vi "battery Profile.vi"() -> ()   [LabVIEW 2015]
uses:
  <instrlib>/Agilent N6700 Series/Agilent N6700 Series.lvlib
panel:
  out "error out 3":errorcluster
  out "error out":errorcluster
  out "Ver":string
  out "error out 2":errorcluster
  in  "Data Log Period (s)":dbl=1.0 format="%#_13g"
  in  "VISA resource name":refnum<visa-resource-name>="VAL_N6705B"
  in  "Number Of DUT":i32=1
  in  "Reset Time (S) \nAfter Discharging":u32
  in  "Number Of Cycle\n(Charching & Discharching For Each DUT":i32=1
  in  "Test Machine IP":string="192.168.1.200"
  in  "Stop":bool
  out "Control Value:Get All":cluster{"Name":string, "Variant Data":variant}[](array[cluster])
  in  "Save":bool
  in  "Start":bool
  out "Status":string
  out "Time 2":dbl caption="Time(s)" format="%#.0f"
  in  "Sleep (s)":u32=3000
  out "Curent Tracking 2":dbl caption="Curent Tracking" format="%.8f"
  out "Voltage Tracking 2":dbl caption="Voltage Tracking" format="%.8f"
  in  "Discharge Stop Voltage":dbl=3.5 format="%#_13g"
  in  "Discharg current Limit":dbl=-0.1 format="%#_13f"
  out "Charging P 2":bool
  out "Charging P 1":bool
  out "Time(s)":u64
  in  "Stop Current(A) after Full":dbl=0.05 format="%#_13g"
  out "Current Tracking":dbl format="%.8f"
  out "Voltage Tracking":dbl format="%.8f"
  in  "Stop Voltage(V)":dbl=4.34 format="%_5f"
  in  "Charge Current (A)":dbl=0.06 format="%#_13g"
  in  "Set Voltge(V)":dbl=4.35 format="%_3f"
  # "Battery Tester"
  # "Battery Charging"
  # "Battery Discharging"
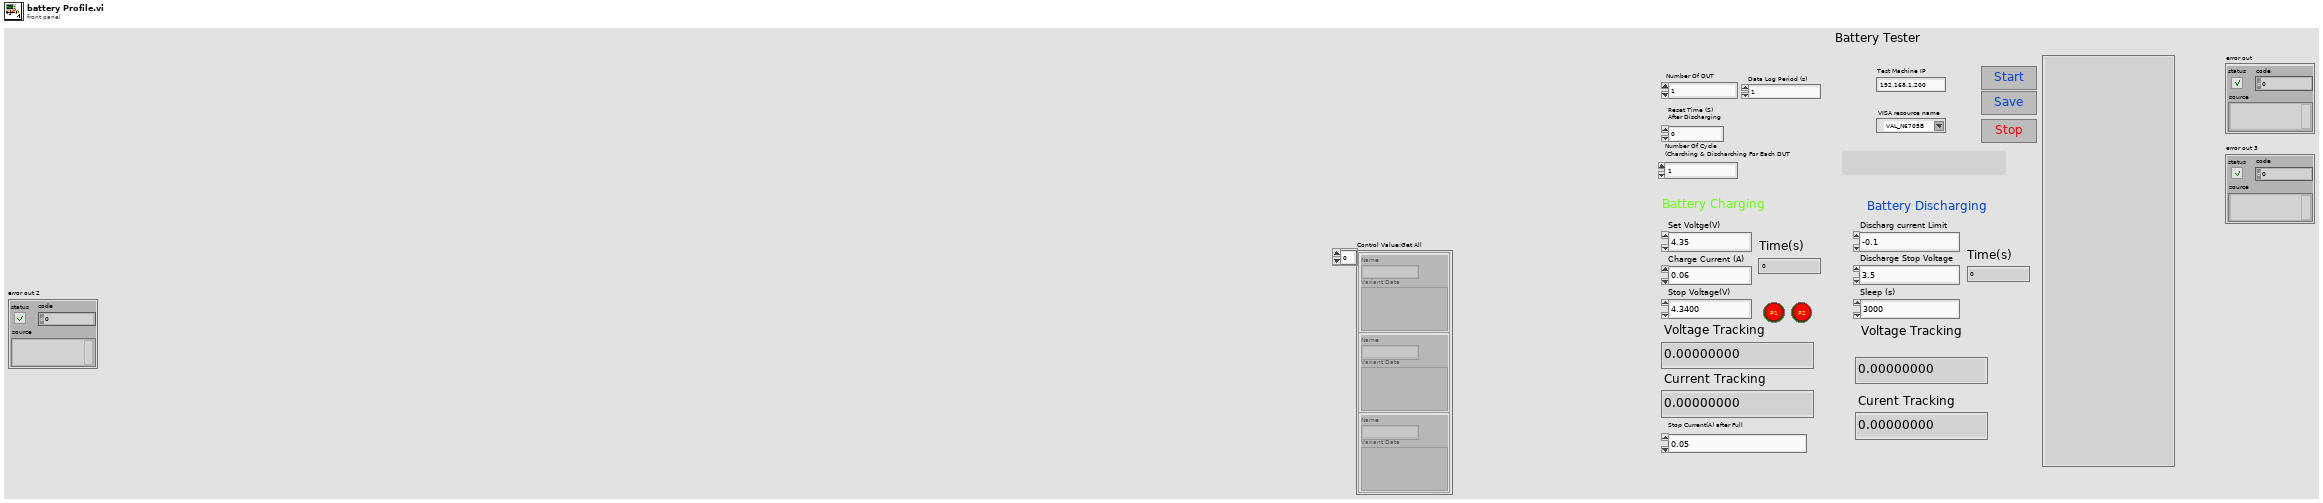
[diagram p1: front panel]
types:
  T1 = enum16{"2 Quad Power Supply", "Unipower Supply", "CC Load", "CV Load", "VM", "CM"}
  T2 = enum16{"open", "replace", "create", "open or create", "replace or create", "replace or create with confirmation"}
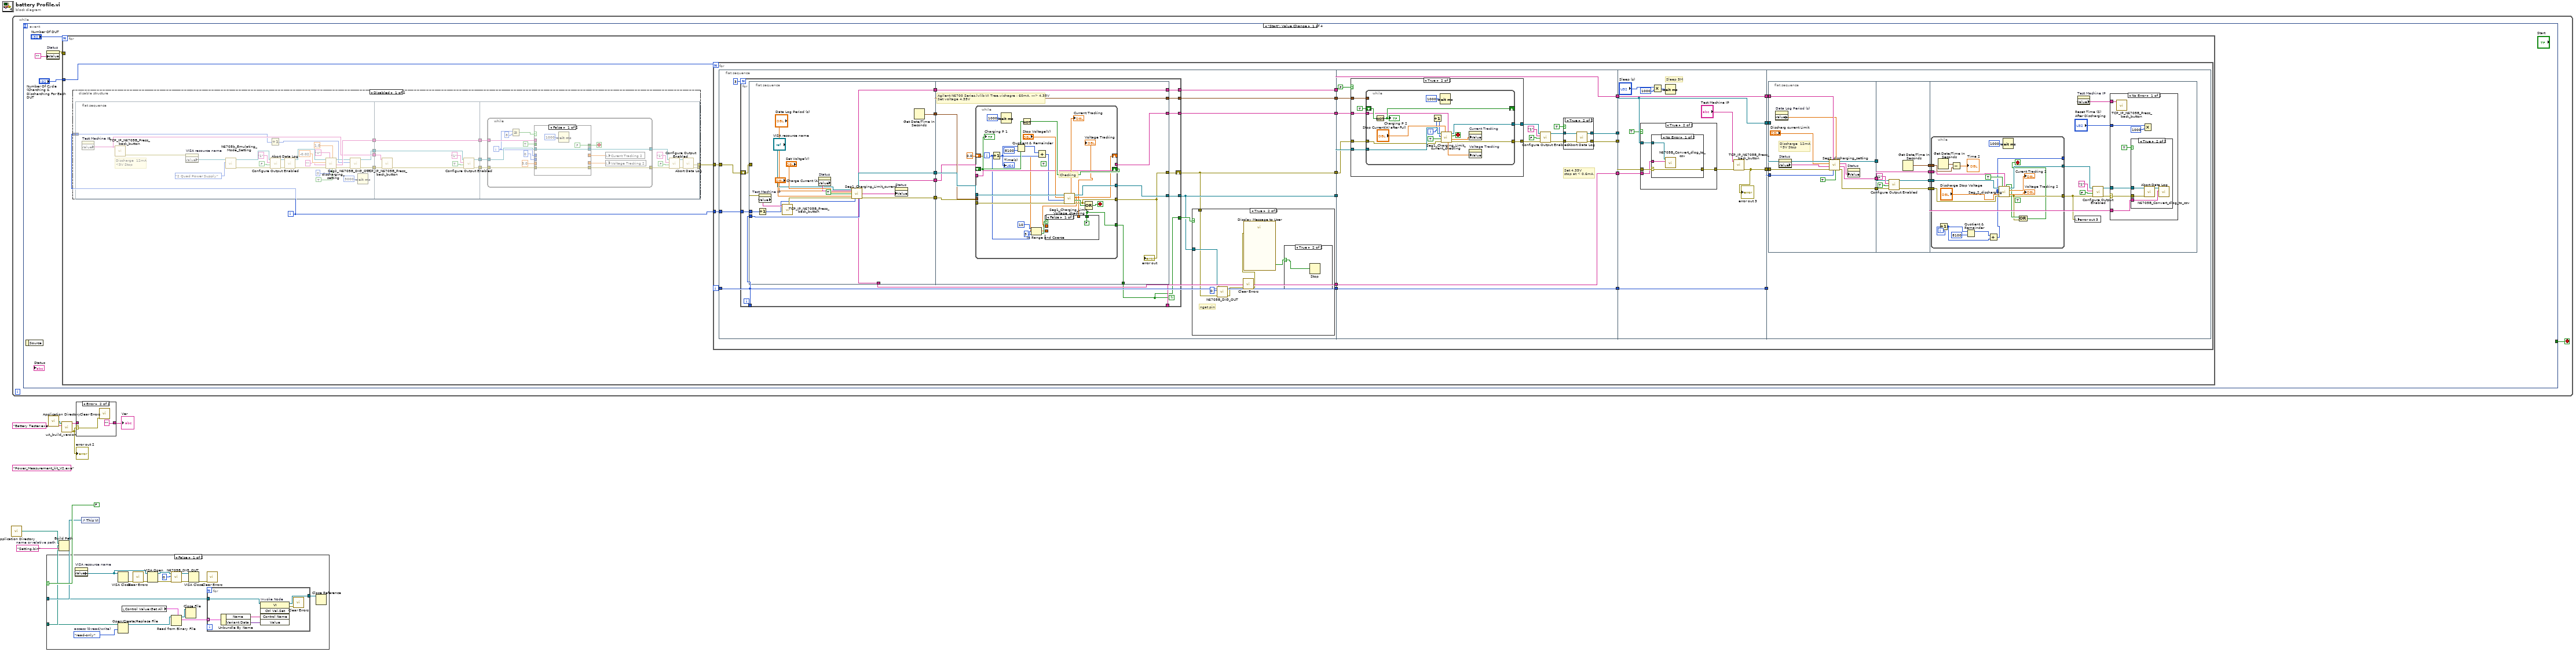
[diagram p0: block diagram]
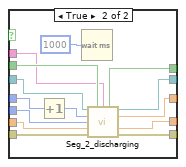
[diagram p3: hidden frame]
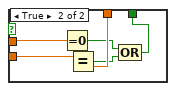
[diagram p7: hidden frame]
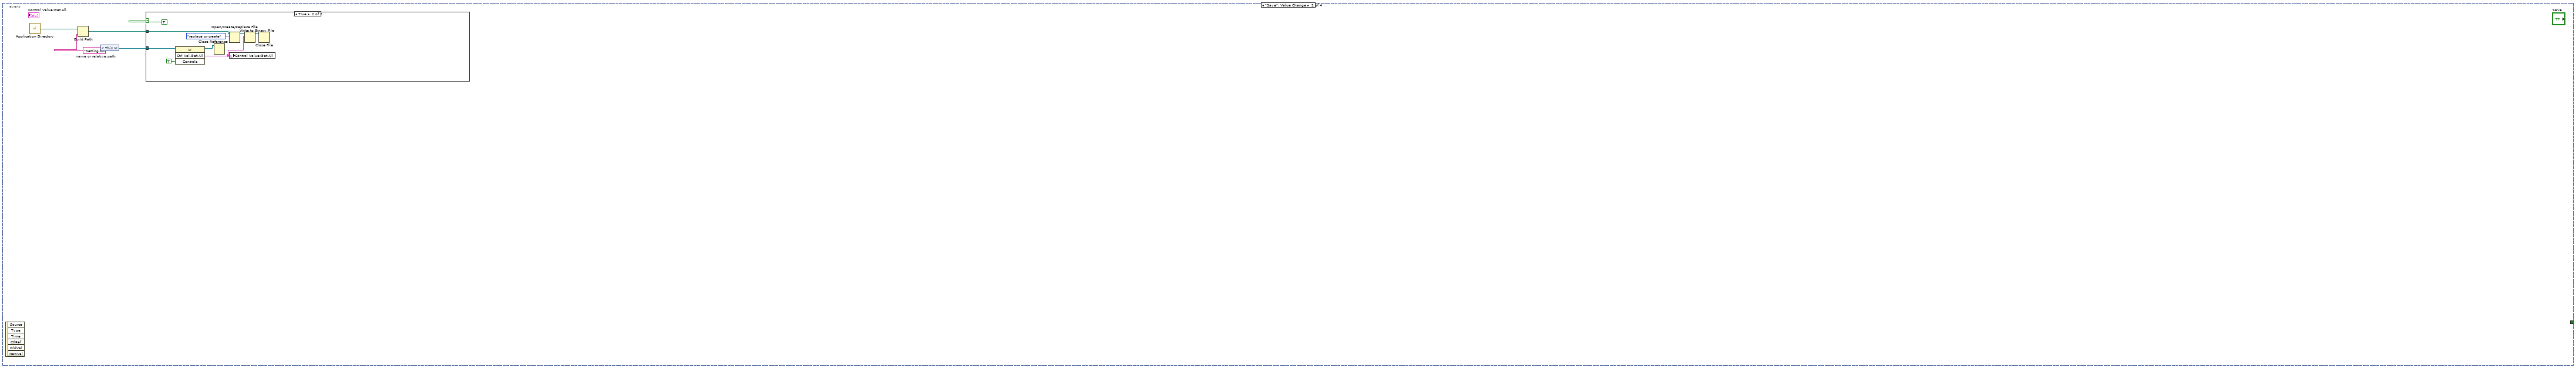
[diagram p14: hidden frame]
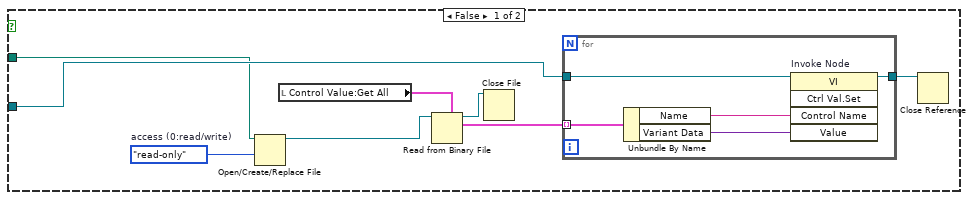
[diagram p15: hidden frame]
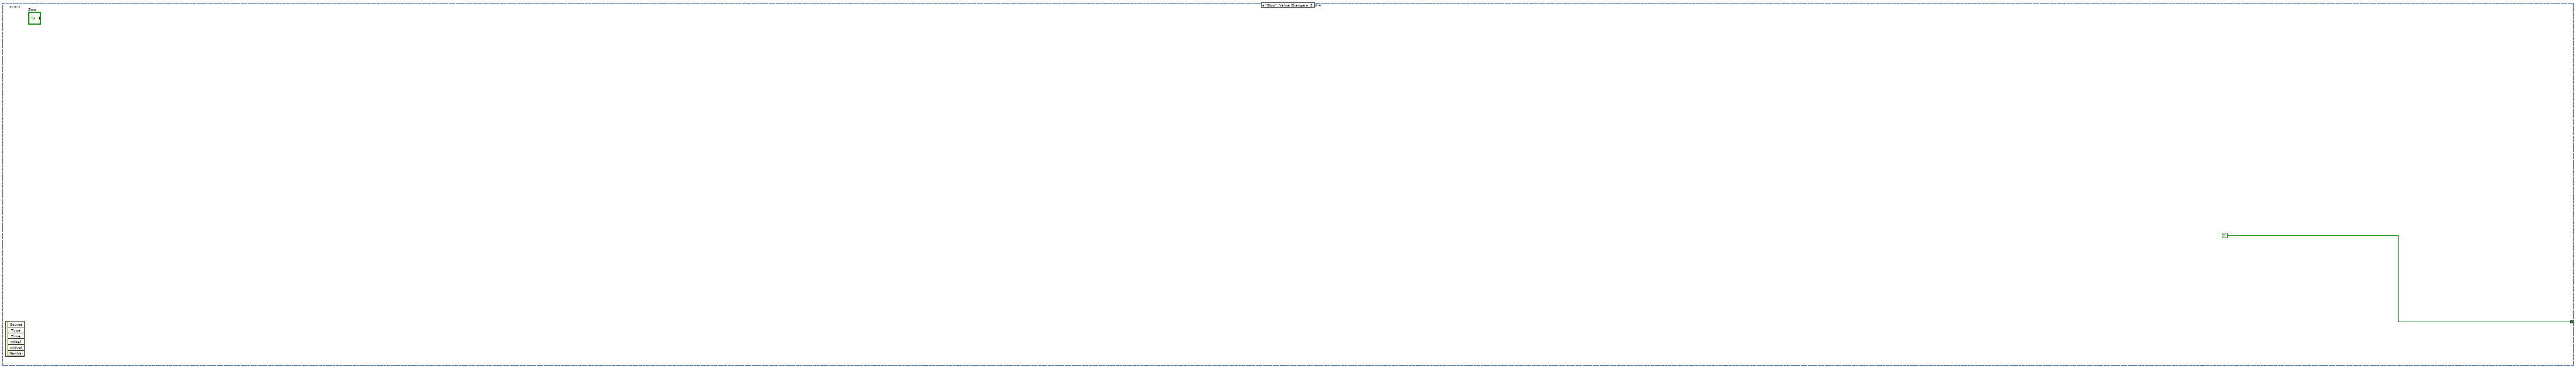
[diagram p16: hidden frame]
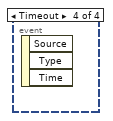
[diagram p17: hidden frame]
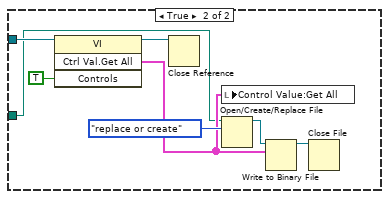
[diagram p18: hidden frame]
diagram:
  (unwired) "Power_Measurement_kit_V2.exe" ("name or relative path")
  w7 = "Setting.bin"  # name or relative path
  n1 = call <vilib>:"Application Directory.vi"() -> ("Application Directory"=w8:path)
  n2 = while {
    stop <- w11 stop-if-true
    n3 = event shown="[0] \"Start\": Value Change" {
      selector: _ -> [_ _ _ _]
      dyn-events: _ -> [_ _ _ _]
      timeout: _ -> [_ _ _ _]
      tunnel: [_ _ TRUE _] -> w11
      event "Start": Value Change {
        n4 = event-data() -> ()  [unwired: 1 in, 1 out]
        n5 = property on="Status" class="Str"("Value"="") -> (error out=w12:errorcluster)  [unwired: 2 in, 1 out]
        n6 = for {
          N: "Number Of DUT" -> [_]
          tunnel: "Number Of Cycle\n(Charching & Discharching For Each DUT" -> [w18]
          tunnel: w12 -> [_]
          i -> [w16]
          n7 = disable-structure shown="Disabled" {
            disable-tunnel: [w20 _] -> w17
            disable-tunnel: w16 -> [w19 _]
            frame Disabled {
              n8 = flat-sequence {
                tunnel: [w32] -> w27
                tunnel: [w31] -> w26
                tunnel: [w52] -> w25
                tunnel: [w34] -> w24
                tunnel: w19 -> [w28]
                tunnel: w27 -> [w60]
                tunnel: w26 -> [w55]
                tunnel: [w59] -> w23
                tunnel: [w58] -> w22
                tunnel: w25 -> [w57]
                tunnel: [w57] -> w21
                tunnel: w24 -> [w54]
                tunnel: w23 -> [w72]
                tunnel: w22 -> [w71]
                tunnel: w21 -> [w65]
                tunnel: [w64] -> w20
                frame #0 {
                  # "Discharge  12mA\n<3V Stop"
                  n9 = property on="Test Machine IP" class="Str"() -> ("Value"=w34:string)  [unwired: 2 in, 2 out]
                  n10 = call "TCP_IP_N6705B_Press_back_button.vi"("instrument address"=w34) -> ("error out"=w46:errorcluster)  [unwired: 10 in]
                  n11 = property on="VISA resource name" class="VISAName"(error in=w46) -> ("Value"=w49:refnum<visa-resource-name>)  [unwired: 1 in, 2 out]
                  n12 = call "N6705b_Emulating_Mode_Setting.vi"("Mode"=T1."2 Quad Power Supply", "VISA resource name"=w49) -> ("error out"=w42:errorcluster, "VISA resource name out"=w44:refnum<visa-resource-name>)  [unwired: 8 in]
                  n13 = Increment(x=w28) -> (x+1=w29:i32)
                  n14 = call <instrlib>:"Configure Output Enabled.vi"("error in (no error)"=w42, "Enable Output (False)"=FALSE, "Channel Name (1)"="1", "VISA resource name"=w44) -> ("error out"=w41:errorcluster, "VISA resource name out"=w43:refnum<visa-resource-name>)  [unwired: 6 in]
                  n15 = call <instrlib>:"Abort Data Log.vi"("error in (no error)"=w41, "VISA resource name"=w43) -> ("error out"=w35:errorcluster, "VISA resource name out"=w45:refnum<visa-resource-name>)  [unwired: 8 in]
                  n16 = call "Seg2_discharging_setting.vi"("Log?"=TRUE, "Data Log Period (0.1 s)"=1.0, "Number of cycles"=0, "N"="X", "error in (no error)"=w35, "Value"="", "Discharg current Limit"=-0.02 ("Discharg current Limit 2"), "VISA Refnum in"=w45) -> ("error out"=w30:errorcluster, "File Name Out"=w52:string, "VISA Refnum out"=w33:refnum<visa-resource-name>)  [unwired: 1 out]
                  n17 = call "N6705B_DIG_OUT.vi"("error in (no error)"=w30, "DUT_1_4"=w29, "VISA Refnum in"=w33) -> ("error out"=w31:errorcluster, "VISA Refnum out"=w32:refnum<visa-resource-name>)  [unwired: 7 in]
                  n18 = Wait (ms)(milliseconds to wait=u32 3000) -> ()  [unwired: 1 out]
                }
                frame #1 {
                  n19 = call "TCP_IP_N6705B_Press_back_button.vi"("error in (no error)"=w55, "instrument address"=w54) -> ("error out"=w56:errorcluster)  [unwired: 9 in]
                  n20 = call <instrlib>:"Configure Output Enabled.vi"("error in (no error)"=w56, "Enable Output (False)"=TRUE, "Channel Name (1)"="1", "VISA resource name"=w60) -> ("error out"=w58:errorcluster, "VISA resource name out"=w59:refnum<visa-resource-name>)  [unwired: 6 in]
                }
                frame #2 {
                  n21 = while {
                    tunnel: w72 -> [w86]
                    tunnel: w71 -> [w85]
                    tunnel: [w84] -> w67
                    tunnel: w65 -> [w80]
                    tunnel: [w73] -> w63
                    i -> [w77]
                    stop <- w83 stop-if-true
                    n22 = Greater Or Equal?(x=w77, y=8) -> (x >= y?=w76:bool)
                    n23 = case shown="False" w76 {
                      tunnel: w86 -> [w89 w104]
                      tunnel: w85 -> [w90 w103]
                      tunnel: [w89 w102] -> w84
                      tunnel: [FALSE ("Stop discharging") w101] -> w83
                      tunnel: 3.0 ("Discharge Stop Voltage 2") -> [_ w100]
                      tunnel: TRUE ("Log??") -> [_ w99]
                      tunnel: w80 -> [_ w98]
                      tunnel: [_ w97] -> w79
                      tunnel: [w90 w96] -> w73
                      tunnel: w77 -> [_ w93]
                      tunnel: 0 ("Index") -> [_ w95]
                      tunnel: [_ w94] -> w74
                      frame False {
                        n24 = Wait (ms)(milliseconds to wait=u32 1000) -> ()  [unwired: 1 out]
                      }
                      frame True {
                        n25 = Increment(x=w93) -> (x+1=w92:i32)
                        n26 = Wait (ms)(milliseconds to wait=u32 1000) -> ()  [unwired: 1 out]
                        n27 = call "Seg_2_discharging.vi"("VISA Refnum in"=w104, "Log??"=w99, "File_name"=w98, "Numeric"=w92, "Index"=w95, "Discharge Stop Voltage"=w100, "error in (no error)"=w103) -> ("Stop discharging"=w101:bool, "VISA Refnum out"=w102:refnum<visa-resource-name>, "Curent Tracking 2"=w94:dbl, "Voltage Tracking 2"=w97:dbl, "error out"=w96:errorcluster)  [unwired: 4 in]
                      }
                    }
                    n28 = local write "Curent Tracking 2"(w74) -> ()
                    n29 = local write "Voltage Tracking 2"(w79) -> ()
                  }
                  n30 = call <instrlib>:"Configure Output Enabled.vi"("error in (no error)"=w63, "Enable Output (False)"=FALSE, "Channel Name (1)"="1", "VISA resource name"=w67) -> ("error out"=w66:errorcluster, "VISA resource name out"=w68:refnum<visa-resource-name>)  [unwired: 6 in]
                  n31 = call <instrlib>:"Abort Data Log.vi"("error in (no error)"=w66, "VISA resource name"=w68) -> ("error out"=w64:errorcluster)  [unwired: 8 in, 1 out]
                }
              }
            }
            frame Enabled {
            }
          }
          n32 = for {
            N: w18 -> [_]
            tunnel: w16 -> [w114]
            tunnel: w17 -> [w106]
            i -> [w112]
            n33 = flat-sequence {
              tunnel: [w125] -> w123
              tunnel: [w124] -> w122
              tunnel: [w134] -> w121
              tunnel: [w133] -> w120
              tunnel: w114 -> [w132]
              tunnel: w112 -> [w131]
              tunnel: [w131] -> w111
              tunnel: [w130] -> w108
              tunnel: w106 -> [w129]
              tunnel: [w128] -> w105
              tunnel: w123 -> [w231]
              tunnel: w122 -> [w230]
              tunnel: [w224] -> w119
              tunnel: [w223] -> w118
              tunnel: w121 -> [w222]
              tunnel: w120 -> [w221]
              tunnel: [w221] -> w117
              tunnel: w111 -> [w219]
              tunnel: [w219] -> w109
              tunnel: w108 -> [w218]
              tunnel: [w218] -> w107
              tunnel: w105 -> [w215]
              tunnel: [w265] -> w116
              tunnel: w119 -> [w265]
              tunnel: w118 -> [w268]
              tunnel: [w270] -> w115
              tunnel: w117 -> [w270]
              tunnel: [w262] -> w113
              tunnel: [w266] -> w110
              tunnel: w109 -> [w266]
              tunnel: w107 -> [w264]
              tunnel: w116 -> [w293]
              tunnel: w115 -> [w287]
              tunnel: w113 -> [w286]
              tunnel: w110 -> [w285]
              frame #0 {
                n34 = for {
                  N: 3 -> [_]
                  tunnel: [w151] -> w125
                  tunnel: [w149] -> w134
                  tunnel: [w148] -> w133
                  tunnel: w132 -> [w147]
                  tunnel: w131 -> [w146]
                  tunnel: [w145] -> w130
                  tunnel: [w143] -> w128
                  shift-right: [w150] -> w124
                  shift-left: w129 -> [w144]
                  tunnel: [w142] -> w126
                  stop <- w142 continue-if-true
                  n35 = flat-sequence {
                    tunnel: [w173] -> w156
                    tunnel: [w172] -> w155
                    tunnel: [w170] -> w154
                    tunnel: [w166] -> w153
                    tunnel: w147 -> [w163]
                    tunnel: w146 -> [w160]
                    tunnel: [w158] -> w145
                    tunnel: [w158] -> w152
                    tunnel: w144 -> [w157]
                    tunnel: w156 -> [w184]
                    tunnel: w155 -> [w183]
                    tunnel: [w182] -> w151
                    tunnel: [w178] -> w150
                    tunnel: w154 -> [w181]
                    tunnel: [w181] -> w149
                    tunnel: w153 -> [w180]
                    tunnel: [w180] -> w148
                    tunnel: w152 -> [w179]
                    tunnel: [w177] -> w143
                    tunnel: [w176] -> w142
                    frame #0 {
                      n36 = Increment(x=w163) -> (x+1=w162:i32)
                      n37 = property on="Test Machine IP" class="Str"(error in=w157) -> ("Value"=w165:string)  [unwired: 1 in, 2 out]
                      n38 = call "TCP_IP_N6705B_Press_back_button.vi"("instrument address"=w165) -> ("error out"=w164:errorcluster)  [unwired: 10 in]
                      n39 = property on="Status" class="Str"() -> ("Value"=w169:string)  [unwired: 2 in, 2 out]
                      n40 = call "Seg1_Charging_Limit_current.vi"("VISA Refnum in"="VISA resource name", "Value"=w169, "Data Log Period (0.1 s)"="Data Log Period (s)", "Set Voltge(V)"="Set Voltge(V)", "Log?"=TRUE, "Charge Current (A)"="Charge Current (A)", "error in (no error)"=w164, "Numeric"=w162, "Number of cycles"=w160) -> ("VISA Refnum out"=w173:refnum<visa-resource-name>, "String"=w166:string, "File Name Out"=w158:string, "String 2"=w168:string, "error out"=w172:errorcluster)  [unwired: 2 in]
                      n41 = property on="Status" class="Str"("Value"=w168) -> ()  [unwired: 2 in, 2 out]
                      n42 = Get Date/Time In Seconds() -> (seconds since 1Jan1904=w170:timestamp)
                    }
                    frame #1 {
                      # "Agilent N6700 Series.lvlib:VI Tree.vichagre : 60mA, ---> 4.35V\nSet voltage 4.35V"
                      n43 = while {
                        tunnel: w184 -> [w207]
                        tunnel: w183 -> [w206]
                        tunnel: [w205] -> w182
                        tunnel: [w195] -> w178
                        tunnel: w181 -> [_]
                        shift-right: [w202] -> _
                        shift-left: _ -> [w203]
                        tunnel: w179 -> [w193]
                        tunnel: [w193] -> w177
                        tunnel: [w185] -> w176
                        shift-right: [w186] -> _
                        shift-left: 0.0 ("Voltage Tracking") -> [w187]
                        i -> [w188]
                        stop <- w194 stop-if-true
                        (unwired) TRUE ("Log?")
                        # "Checking"
                        n44 = Increment(x=w188) -> (x+1=w197:i32)
                        "Time(s)" <- w197
                        n45 = Wait (ms)(milliseconds to wait=u32 1000) -> ()  [unwired: 1 out]
                        n46 = Quotient & Remainder(x=w197, y=8100) -> (x-y*floor(x/y)=w198:i32)  [unwired: 1 out]
                        n47 = Not(x=w203) -> (.not. x?=w202:bool)
                        n48 = In Range and Coerce(upper limit=10 ("y"), x=w188, lower limit=3) -> (In Range?=w189:bool)  [unwired: 1 out]
                        n49 = Add(x=w198, y=w197) -> (x+y=w192:i32)
                        n50 = call "Seg1_Charging_Limit_Voltage_checking.vi"("error in (no error)"=w206, "Numeric"=w192, "Stop Voltage(V)"="Stop Voltage(V)", "VISA Refnum in"=w207) -> ("error out"=w195:errorcluster, "Boolean"=w196:bool, "Voltage Tracking"=w186:dbl, "VISA Refnum out"=w205:refnum<visa-resource-name>, "Current Tracking"=→"Current Tracking":dbl)  [unwired: 3 in]
                        "Voltage Tracking" <- w186
                        n51 = case shown="False" w189 {
                          tunnel: w186 -> [_ w214]
                          tunnel: w187 -> [_ w213]
                          tunnel: w186 -> [_ w212]
                          tunnel: [FALSE w209] -> w185
                          frame False {
                          }
                          frame True {
                            n52 = Equal To 0?(x=w214) -> (x = 0?=w211:bool)
                            n53 = Equal?(x=w213, y=w212) -> (x = y?=w210:bool)
                            n54 = Compound Arithmetic op=OR(w211, w210) -> (w209:bool)
                          }
                        }
                        n55 = Compound Arithmetic op=OR(w195, w196, w185) -> (w194:bool)
                        "Charging P 1" <- w203
                      }
                      "error out" <- w178
                    }
                  }
                }
                n56 = case shown="True" w126 {
                  tunnel: w125 -> [_ w140]
                  tunnel: w124 -> [_ w138]
                  frame False {
                  }
                  frame True {
                    # "ngat pin"
                    n57 = call "N6705B_DIG_OUT.vi"("error in (no error)"=w138, "DUT_1_4"=0, "VISA Refnum in"=w140) -> ("error out"=w139:errorcluster)  [unwired: 7 in, 1 out]
                    n58 = call <vilib>:"Clear Errors.vi"("error in (no error)"=w139) -> ("error out"=w136:errorcluster)  [unwired: 5 in, 1 out]
                    n59 = call "Display Message to User"("error in (no error)"=w136) -> ("OK"=w135:bool)  [unwired: 9 in, 1 out]
                    n60 = case shown="True" w135 {
                      selector: w135 -> [_ w141]
                      frame False {
                      }
                      frame True {
                        n61 = Stop(stop? (T)=w141) -> ()
                      }
                    }
                  }
                }
              }
              frame #1 {
                # "Set 4.35V\nstop at < 0.6mA,"
                n62 = case shown="True" FALSE {
                  tunnel: w231 -> [w239 w246]
                  tunnel: w230 -> [w238 w245]
                  tunnel: [w239 w244] -> w228
                  tunnel: [w238 w243] -> w227
                  tunnel: w222 -> [_ w242]
                  tunnel: w215 -> [_ w240]
                  frame False {
                    # "Anh Nguyen Request Jan 01 2018"
                  }
                  frame True {
                    n63 = while {
                      tunnel: w246 -> [w261]
                      tunnel: w245 -> [w260]
                      tunnel: [w254] -> w244
                      tunnel: [w251] -> w243
                      tunnel: w242 -> [_]
                      shift-right: [w255] -> _
                      shift-left: TRUE -> [w256]
                      tunnel: w240 -> [w247]
                      i -> [w249]
                      stop <- w259 stop-if-true
                      n64 = Not(x=w256) -> (.not. x?=w255:bool)
                      "Charging P 2" <- w255
                      n65 = Increment(x=w249) -> (x+1=w248:i32)
                      n66 = Wait (ms)(milliseconds to wait=u32 1000) -> ()  [unwired: 1 out]
                      n67 = call "Seg1_Charging_Limit_current_checking.vi"("File_name"=w247, "Stop Current(A) after Full"="Stop Current(A) after Full", "error in (no error)"=w260, "Log?"=TRUE, "Numeric 3"=w248, "VISA Refnum in"=w261) -> ("error out"=w251:errorcluster, "Peak to Peak 2 (Curr)"=w257:dbl, "Boolean"=w259:bool, "VISA Refnum out"=w254:refnum<visa-resource-name>, "Peak to Peak (vol)"=w253:dbl)  [unwired: 1 in]
                      n68 = property on="Current Tracking" class="DigNum (strict)"("Value"=w257) -> ()  [unwired: 2 in, 2 out]
                      n69 = property on="Voltage Tracking" class="DigNum (strict)"("Value"=w253) -> ()  [unwired: 2 in, 2 out]
                    }
                  }
                }
                n70 = call <instrlib>:"Configure Output Enabled.vi"("error in (no error)"=w227, "Enable Output (False)"=FALSE, "Channel Name (1)"="1", "VISA resource name"=w228) -> ("error out"=w217:errorcluster, "VISA resource name out"=w226:refnum<visa-resource-name>)  [unwired: 6 in]
                n71 = case shown="True" TRUE {
                  tunnel: w226 -> [w233 w237]
                  tunnel: [w233 w236] -> w224
                  tunnel: [w232 w235] -> w223
                  tunnel: w217 -> [w232 w234]
                  frame False {
                  }
                  frame True {
                    n72 = call <instrlib>:"Abort Data Log.vi"("error in (no error)"=w234, "VISA resource name"=w237) -> ("error out"=w235:errorcluster, "VISA resource name out"=w236:refnum<visa-resource-name>)  [unwired: 8 in]
                  }
                }
              }
              frame #2 {
                # "Sleep 5M"
                n73 = case shown="True" TRUE {
                  tunnel: w268 -> [w274 w278]
                  tunnel: [w274 w277] -> w267
                  tunnel: w265 -> [_ w276]
                  tunnel: w264 -> [_ w275]
                  frame False {
                  }
                  frame True {
                    n74 = case shown="No Error" w278 {
                      selector: w278 -> [w281 w282]
                      tunnel: [w281 w282] -> w277
                      tunnel: w276 -> [w280 _]
                      tunnel: w275 -> [w279 _]
                      frame No Error {
                        n75 = call "N6705B_Convert_dlog_to_csv.vi"("File Name Out"=w279, "VISA Refnum in"=w280) -> ()  [unwired: 10 in]
                      }
                      frame Error {
                      }
                    }
                  }
                }
                n76 = Multiply(x="Sleep (s)", y=u32 1000) -> (x*y=w272:u32)
                n77 = Wait (ms)(milliseconds to wait=w272) -> ()  [unwired: 1 out]
                n78 = call "TCP_IP_N6705B_Press_back_button.vi"("error in (no error)"=w267, "instrument address"="Test Machine IP") -> ("error out"=w262:errorcluster)  [unwired: 9 in]
                "error out 3" <- w262
              }
              frame #3 {
                n79 = flat-sequence {
                  tunnel: w293 -> [w305]
                  tunnel: [w303] -> w292
                  tunnel: [w302] -> w291
                  tunnel: w287 -> [w299]
                  tunnel: w286 -> [w298]
                  tunnel: w285 -> [w296]
                  tunnel: [w295] -> w284
                  tunnel: w292 -> [w311]
                  tunnel: w291 -> [w310]
                  tunnel: [w309] -> w290
                  tunnel: [w308] -> w289
                  tunnel: [w307] -> w288
                  tunnel: w284 -> [w306]
                  tunnel: [w306] -> w283
                  tunnel: w290 -> [w325]
                  tunnel: w289 -> [w324]
                  tunnel: w288 -> [w323]
                  tunnel: w283 -> [w315]
                  frame #0 {
                    # "Discharge  12mA\n<3V Stop"
                    n80 = property on="Data Log Period (s)" class="DigNum (strict)"() -> ("Value"=w297:dbl)  [unwired: 2 in, 2 out]
                    n81 = property on="Status" class="Str"() -> ("Value"=w301:string)  [unwired: 2 in, 2 out]
                    n82 = call "Seg2_discharging_setting.vi"("Log?"=TRUE, "Data Log Period (0.1 s)"=w297, "Number of cycles"=w296, "N"=w299, "error in (no error)"=w298, "Value"=w301, "Discharg current Limit"="Discharg current Limit", "VISA Refnum in"=w305) -> ("error out"=w302:errorcluster, "File Name Out"=w295:string, "String out"=w300:string, "VISA Refnum out"=w303:refnum<visa-resource-name>)
                    n83 = property on="Status" class="Str"("Value"=w300) -> ()  [unwired: 2 in, 2 out]
                  }
                  frame #1 {
                    n84 = call <instrlib>:"Configure Output Enabled.vi"("error in (no error)"=w310, "Enable Output (False)"=TRUE, "Channel Name (1)"="1", "VISA resource name"=w311) -> ("error out"=w308:errorcluster, "VISA resource name out"=w309:refnum<visa-resource-name>)  [unwired: 6 in]
                    n85 = Get Date/Time In Seconds() -> (seconds since 1Jan1904=w307:timestamp)
                  }
                  frame #2 {
                    n86 = while {
                      tunnel: w325 -> [w356]
                      tunnel: w324 -> [w355]
                      tunnel: [w354] -> w317
                      tunnel: [w338] -> w314
                      tunnel: [w340] -> _
                      tunnel: w323 -> [w352]
                      tunnel: w315 -> [w346]
                      i -> [w344]
                      stop <- w337 stop-if-true
                      (unwired) TRUE ("Log?")
                      n87 = Get Date/Time In Seconds() -> (seconds since 1Jan1904=w353:timestamp)
                      n88 = Increment(x=w344) -> (x+1=w341:i32)
                      n89 = Subtract(x=w353, y=w352) -> (x-y=→"Time 2":dbl)
                      n90 = Quotient & Remainder(x=w341, y=8100) -> (x-y*floor(x/y)=w343:i32)  [unwired: 1 out]
                      n91 = Add(x=w343, y=w341) -> (x+y=w340:i32)
                      n92 = call "Seg_2_discharging.vi"("VISA Refnum in"=w356, "Log??"=TRUE, "File_name"=w346, "Numeric"=w340, "Index"=w340, "Discharge Stop Voltage"="Discharge Stop Voltage", "error in (no error)"=w355) -> ("Stop discharging"=w339:bool, "VISA Refnum out"=w354:refnum<visa-resource-name>, "Curent Tracking 2"=→"Curent Tracking 2":dbl, "Voltage Tracking 2"=→"Voltage Tracking 2":dbl, "error out"=w338:errorcluster)  [unwired: 4 in]
                      n93 = Wait (ms)(milliseconds to wait=u32 1000) -> ()  [unwired: 1 out]
                      n94 = Compound Arithmetic op=OR(w339, w338) -> (w337:bool)
                    }
                    n95 = local write "error out 3"(w314) -> ()
                    n96 = property on="Test Machine IP" class="Str"() -> ("Value"=w319:string)  [unwired: 2 in, 2 out]
                    n97 = call <instrlib>:"Configure Output Enabled.vi"("error in (no error)"=w314, "Enable Output (False)"=FALSE, "Channel Name (1)"="1", "VISA resource name"=w317) -> ("error out"=w316:errorcluster, "VISA resource name out"=w318:refnum<visa-resource-name>)  [unwired: 6 in]
                    n98 = case shown="No Error" w316 {
                      selector: w316 -> [w327 _]
                      tunnel: "Reset Time (S) \nAfter Discharging" -> [w332 _]
                      tunnel: w319 -> [w330 _]
                      tunnel: w318 -> [w328 _]
                      tunnel: w315 -> [w329 _]
                      frame No Error {
                        n99 = call "TCP_IP_N6705B_Press_back_button.vi"("instrument address"=w330) -> ()  [unwired: 10 in, 1 out]
                        n100 = case shown="True" TRUE {
                          tunnel: w329 -> [_ w336]
                          tunnel: w328 -> [_ w335]
                          tunnel: w327 -> [_ w333]
                          frame False {
                          }
                          frame True {
                            n101 = call <instrlib>:"Abort Data Log.vi"("error in (no error)"=w333, "VISA resource name"=w335) -> ("VISA resource name out"=w334:refnum<visa-resource-name>)  [unwired: 8 in, 1 out]
                            n102 = call "N6705B_Convert_dlog_to_csv.vi"("File Name Out"=w336, "VISA Refnum in"=w334) -> ()  [unwired: 10 in]
                          }
                        }
                        n103 = Multiply(x=w332, y=u32 1000) -> ()  [unwired: 1 out]
                      }
                      frame Error {
                      }
                    }
                  }
                }
              }
            }
          }
        }
      }
      event "Save": Value Change {
        w358 = "Setting.bin"  # name or relative path
        n104 = event-data() -> ()  [unwired: 1 in, 6 out]
        n105 = call <vilib>:"Application Directory.vi"() -> ("Application Directory"=w359:path)
        n106 = Build Path(base path=w359, name or relative path=w358) -> (appended path=w357:path)
        n107 = control-ref of="This VI"() -> (w360:refnum<vi>)
        n108 = case shown="True" TRUE ("Store Val's When Lit") {
          tunnel: w360 -> [w363 w377]
          tunnel: w357 -> [w362 w375]
          frame False {
            w365 = enum16{"read/write", "read-only", "write-only"}."read-only"  # access (0:read/write)
            n109 = Open/Create/Replace File(file path (use dialog)=w362, access (0:read/write)=w365) -> (refnum out=w366:refnum<file>)  [unwired: 1 in, 5 out]
            n110 = local read "Control Value:Get All"() -> (w368:cluster{"Name":string, "Variant Data":variant}[])
            n111 = Read from Binary File(5:w368, 11:w366) -> (2:w367:cluster{"Name":string, "Variant Data":variant}[], 3:w364:refnum<file>)  [unwired: 1 in, 5 out]
            n112 = Close File(refnum=w364) -> ()  [unwired: 1 in, 2 out]
            n113 = for {
              tunnel: [w374] -> w369
              tunnel: w363 -> [w373]
              tunnel: w367 -> [w372] mode=indexing
              n114 = Unbundle By Name "Unbundle By Name"(w372) -> ("Name"=w371:string, "Variant Data"=w370:variant)
              n115 = invoke on="Invoke Node" class="VI" method="Ctrl Val.Set"(reference=w373, "Control Name"=w371, "Value"=w370) -> (reference out=w374:refnum<vi>)  [unwired: 2 in, 4 out]
            }
            n116 = Close Reference(reference=w369) -> ()  [unwired: 1 in, 1 out]
          }
          frame True {
            n117 = invoke class="VI" method="Ctrl Val.Get All"(reference=w377, "Controls"=TRUE) -> (reference out=w382:refnum<vi>, "Get All Control Values Variant"=w376:cluster{"Name":string, "Variant Data":variant}[])  [unwired: 2 in, 2 out]
            n118 = Close Reference(reference=w382) -> ()  [unwired: 1 in, 1 out]
            n119 = Open/Create/Replace File(file path (use dialog)=w375, operation (0:open)=T2."replace or create") -> (refnum out=w379:refnum<file>)  [unwired: 1 in, 5 out]
            n120 = local write "Control Value:Get All"(w376) -> ()
            n121 = Write to Binary File(file (use dialog)=w379, data=w376) -> (refnum out=w378:refnum<file>)  [unwired: 1 in, 5 out]
            n122 = Close File(refnum=w378) -> ()  [unwired: 1 in, 2 out]
          }
        }
      }
      event "Stop": Value Change {
        n123 = event-data() -> ()  [unwired: 1 in, 6 out]
      }
      event Timeout {
        n124 = event-data() -> ()  [unwired: 1 in, 3 out]
      }
    }
  }
  n125 = call <vilib>:"Application Directory.vi"() -> ("Application Directory"=w5:path)
  n126 = Build Path(base path=w8, name or relative path=w7) -> (appended path=w6:path)
  n127 = call "uA_build_version.vi"("name or relative path"="Battery Tester.exe", "path"=w5) -> ("error out"=w4:errorcluster, "FileVersion"=w3:string)  [unwired: 7 in, 1 out]
  "error out 2" <- w4
  n128 = case shown="Error" w4 {
    selector: w4 -> [_ w386]
    tunnel: w3 -> [w384 _]
    tunnel: [w384 "" ("FileVersion")] -> w2
    frame No Error {
    }
    frame Error {
      n129 = call <vilib>:"Clear Errors.vi"("error in (no error)"=w386) -> ()  [unwired: 5 in, 2 out]
    }
  }
  "Ver" <- w2
  n130 = control-ref of="This VI"() -> (w9:refnum<vi>)
  n131 = case shown="False" FALSE ("Store Val's When Lit") {
    tunnel: w9 -> [w397 w412]
    tunnel: w6 -> [w396 w410]
    frame False {
      w399 = enum16{"read/write", "read-only", "write-only"}."read-only"  # access (0:read/write)
      n132 = property on="VISA resource name" class="VISAName"() -> ("Value"=w389:refnum<visa-resource-name>)  [unwired: 2 in, 2 out]
      n133 = VISA Close(VISA resource name=w389) -> (error out=w391:errorcluster)  [unwired: 1 in]
      n134 = Open/Create/Replace File(file path (use dialog)=w396, access (0:read/write)=w399) -> (refnum out=w400:refnum<file>)  [unwired: 1 in, 5 out]
      n135 = local read "Control Value:Get All"() -> (w402:cluster{"Name":string, "Variant Data":variant}[])
      n136 = call <vilib>:"Clear Errors.vi"("error in (no error)"=w391) -> ("error out"=w390:errorcluster)  [unwired: 5 in, 1 out]
      n137 = VISA Open(error in (no error)=w390, VISA resource name=w389) -> (VISA resource name=w392:refnum<visa-resource-name>, error out=w393:errorcluster)  [unwired: 3 in]
      n138 = call "N6705B_DIG_OUT.vi"("error in (no error)"=w393, "DUT_1_4"=0, "VISA Refnum in"=w392) -> ("error out"=w395:errorcluster, "VISA Refnum out"=w394:refnum<visa-resource-name>)  [unwired: 7 in]
      n139 = Read from Binary File(5:w402, 11:w400) -> (2:w401:cluster{"Name":string, "Variant Data":variant}[], 3:w398:refnum<file>)  [unwired: 1 in, 5 out]
      n140 = Close File(refnum=w398) -> ()  [unwired: 1 in, 2 out]
      n141 = VISA Close(VISA resource name=w394, error in (no error)=w395) -> (error out=w388:errorcluster)
      n142 = call <vilib>:"Clear Errors.vi"("error in (no error)"=w388) -> ()  [unwired: 5 in, 2 out]
      n143 = for {
        tunnel: [w409] -> w403
        tunnel: w397 -> [w408]
        tunnel: w401 -> [w407] mode=indexing
        n144 = Unbundle By Name "Unbundle By Name"(w407) -> ("Name"=w406:string, "Variant Data"=w405:variant)
        n145 = invoke on="Invoke Node" class="VI" method="Ctrl Val.Set"(reference=w408, "Control Name"=w406, "Value"=w405) -> (reference out=w409:refnum<vi>, error out=w404:errorcluster)  [unwired: 2 in, 3 out]
        n146 = call <vilib>:"Clear Errors.vi"("error in (no error)"=w404) -> ()  [unwired: 5 in, 2 out]
      }
      n147 = Close Reference(reference=w403) -> ()  [unwired: 1 in, 1 out]
    }
    frame True {
      n148 = invoke class="VI" method="Ctrl Val.Get All"(reference=w412, "Controls"=TRUE) -> (reference out=w417:refnum<vi>, "Get All Control Values Variant"=w411:cluster{"Name":string, "Variant Data":variant}[])  [unwired: 2 in, 2 out]
      n149 = Close Reference(reference=w417) -> ()  [unwired: 1 in, 1 out]
      n150 = local write "Control Value:Get All"(w411) -> ()
      n151 = Open/Create/Replace File(file path (use dialog)=w410, operation (0:open)=T2."replace or create") -> (refnum out=w414:refnum<file>)  [unwired: 1 in, 5 out]
      n152 = Write to Binary File(file (use dialog)=w414, data=w411) -> (refnum out=w413:refnum<file>)  [unwired: 1 in, 5 out]
      n153 = Close File(refnum=w413) -> ()  [unwired: 1 in, 2 out]
    }
  }
